vi "Get Arg Map.vi"(8 "error in (no error)":errorcluster, 11 "Arguments in":refnum<class "Arguments.lvclass">) -> (0 "error out":errorcluster, 2 "Arguments":map{string, variant}(c390), 3 "Arguments out":refnum<class "Arguments.lvclass">)   [LabVIEW 2020, in "HTTP Server.lvlib" / "Arguments.lvclass"]
uses:
  Arguments.lvclass
  Arguments.lvclass/Arguments.ctl
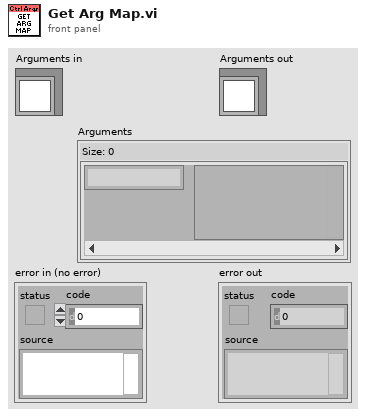
[diagram p1: front panel]
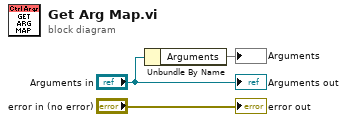
[diagram p0: block diagram]
diagram:
  n1 = Unbundle By Name("Arguments in") -> ("Arguments"=→"Arguments":map{string, variant})
  "error out" <- "error in (no error)"
  "Arguments out" <- "Arguments in"
